vi "comunicacion de labview con excel.vi"() -> ()   [LabVIEW 2013]
panel:
  in  "Path":path
  in  "Knob":dbl(knob) scale=0.0..255.0
  in  "stop":bool
  in  "Guardar":bool
  in  "Power":bool=TRUE
  in  "input 9":string
  in  "timpo de nuestreo":u32
  out "Waveform Chart":dbl(graph)
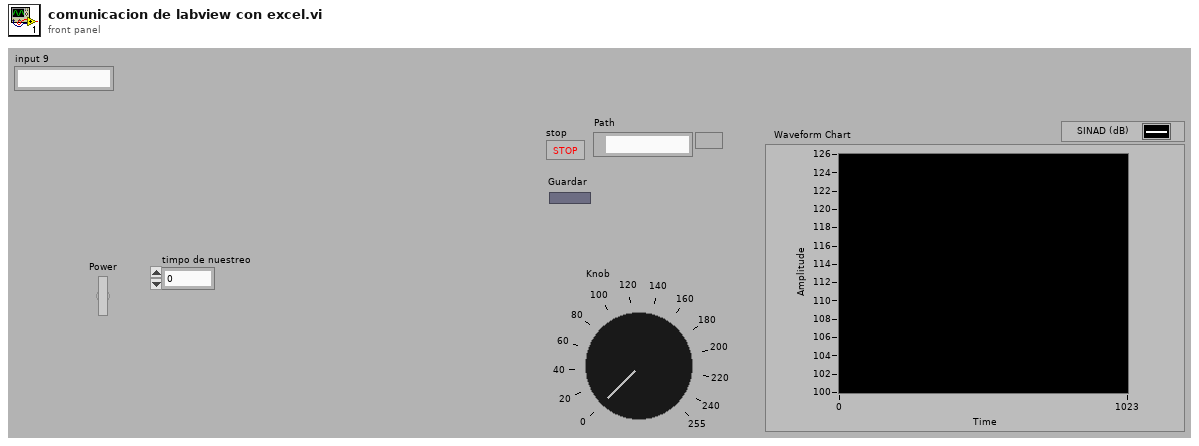
[diagram p1: front panel]
types:
  T1 = enum16{"open", "open or create", "create or replace", "create"}
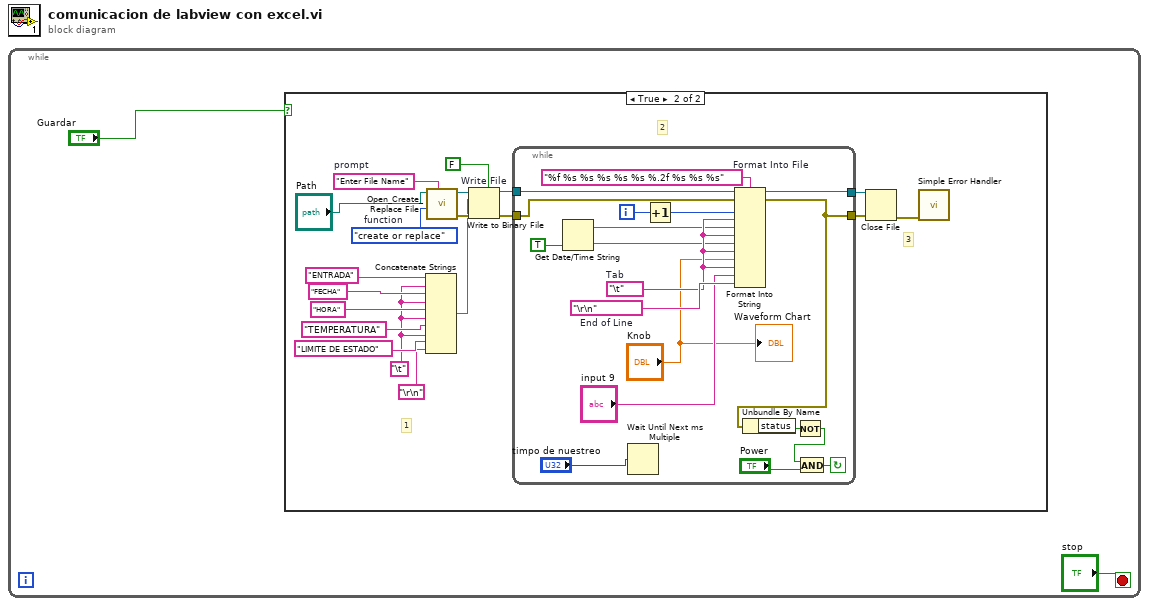
[diagram p0: block diagram]
diagram:
  n1 = while {
    stop <- "stop" stop-if-true
    n2 = case shown="True" "Guardar" {
      frame False {
      }
      frame True {
        w4 = T1."create or replace"  # function
        w9 = "\t"
        w5 = "Enter File Name"  # prompt
        # "1"
        # "3"
        # "2"
        n3 = Concatenate Strings "Concatenate Strings"("ENTRADA", w9, "FECHA", w9, "HORA", w9, "TEMPERATURA", w9, "LIMITE DE ESTADO", "\r\n") -> (w8:string)
        n4 = call <vilib>:"Open_Create_Replace File.vi"("prompt"=w5, "function (open:0)"=w4, "file path"="Path") -> ("error out"=w20:errorcluster, "refnum"=w19:refnum<file>)  [unwired: 3 in, 4 out]
        n5 = Write to Binary File "Write File"(file (use dialog)=w19, data=w8, error in=w20, 5:FALSE ("prepend array or string size? (T)")) -> (refnum out=w7:refnum<file>, error out=w6:errorcluster)  [unwired: 3 out]
        n6 = while {
          tunnel: w6 -> [w36]
          tunnel: w7 -> [w37]
          tunnel: [w32] -> w17
          tunnel: [w37] -> w18
          i -> [w26]
          stop <- w35 continue-if-true
          w31 = "\r\n"  # End of Line
          w30 = "\t"  # Tab
          n7 = Get Date/Time String(want seconds? (F)=TRUE) -> (date string=w27:string, time string=w28:string)  [unwired: 2 out]
          n8 = Wait Until Next ms Multiple(millisecond multiple="timpo de nuestreo") -> ()  [unwired: 1 out]
          n9 = Increment(x=w26) -> (x+1=w23:i32)
          n10 = Format Into String "Format Into File"(format string="%f %s %s %s %s %s %.2f %s %s %s" ("Format String"), initial string=w37, error in=w36, w23, w30, w27, w30, w28, w30, "Knob", w30, "input 9", w31) -> (error out=w32:errorcluster)  [unwired: 1 out]
          n11 = Unbundle By Name(w32) -> ("status"=w33:bool)
          n12 = Not(x=w33) -> (.not. x?=w34:bool)
          n13 = And(x=w34, y="Power") -> (x .and. y?=w35:bool)
          "Waveform Chart" <- "Knob"
        }
        n14 = Close File(refnum=w18, error in=w17) -> (error out=w16:errorcluster)  [unwired: 1 out]
        n15 = call <vilib>:"Simple Error Handler.vi"("error in (no error)"=w16) -> ()  [unwired: 1 in, 8 out]
      }
    }
  }
